vi "Amplifier Output Test Interface.vi"() -> ()   [LabVIEW 2012]
panel:
  out "Power Spectrum / PSD [Filtered]":cluster{"f0":dbl, "df":dbl, "magnitude":dbl[]}(graph)
  out "Signal [Filtered]":waveform(dbl)(graph)
  out "Power Spectrum / PSD [Non Filtered]":cluster{"f0":dbl, "df":dbl, "magnitude":dbl[]}(graph)
  out "Signal [Non Filtered]":waveform(dbl)(graph)
  in  "Filter":T1
  in  "Signal Acquisition":T2 {"Scale Type" items=["Volts"=10348, "Custom Scale"=10065]; "Sample Mode" items=["Finite Samples"=10178, "Continuous Samples"=10123, "Hardware Timed Single Point"=12522]; "Terminal Configuration" items=["Default"=-1, "RSE"=10083, "Differential"=10106, "Pseudodifferential"=12529]}
  in  "error in":errorcluster
  out "error out":errorcluster
  in  "Exit":bool caption="Start 2"
  in  "Filter":bool caption="Start 2"
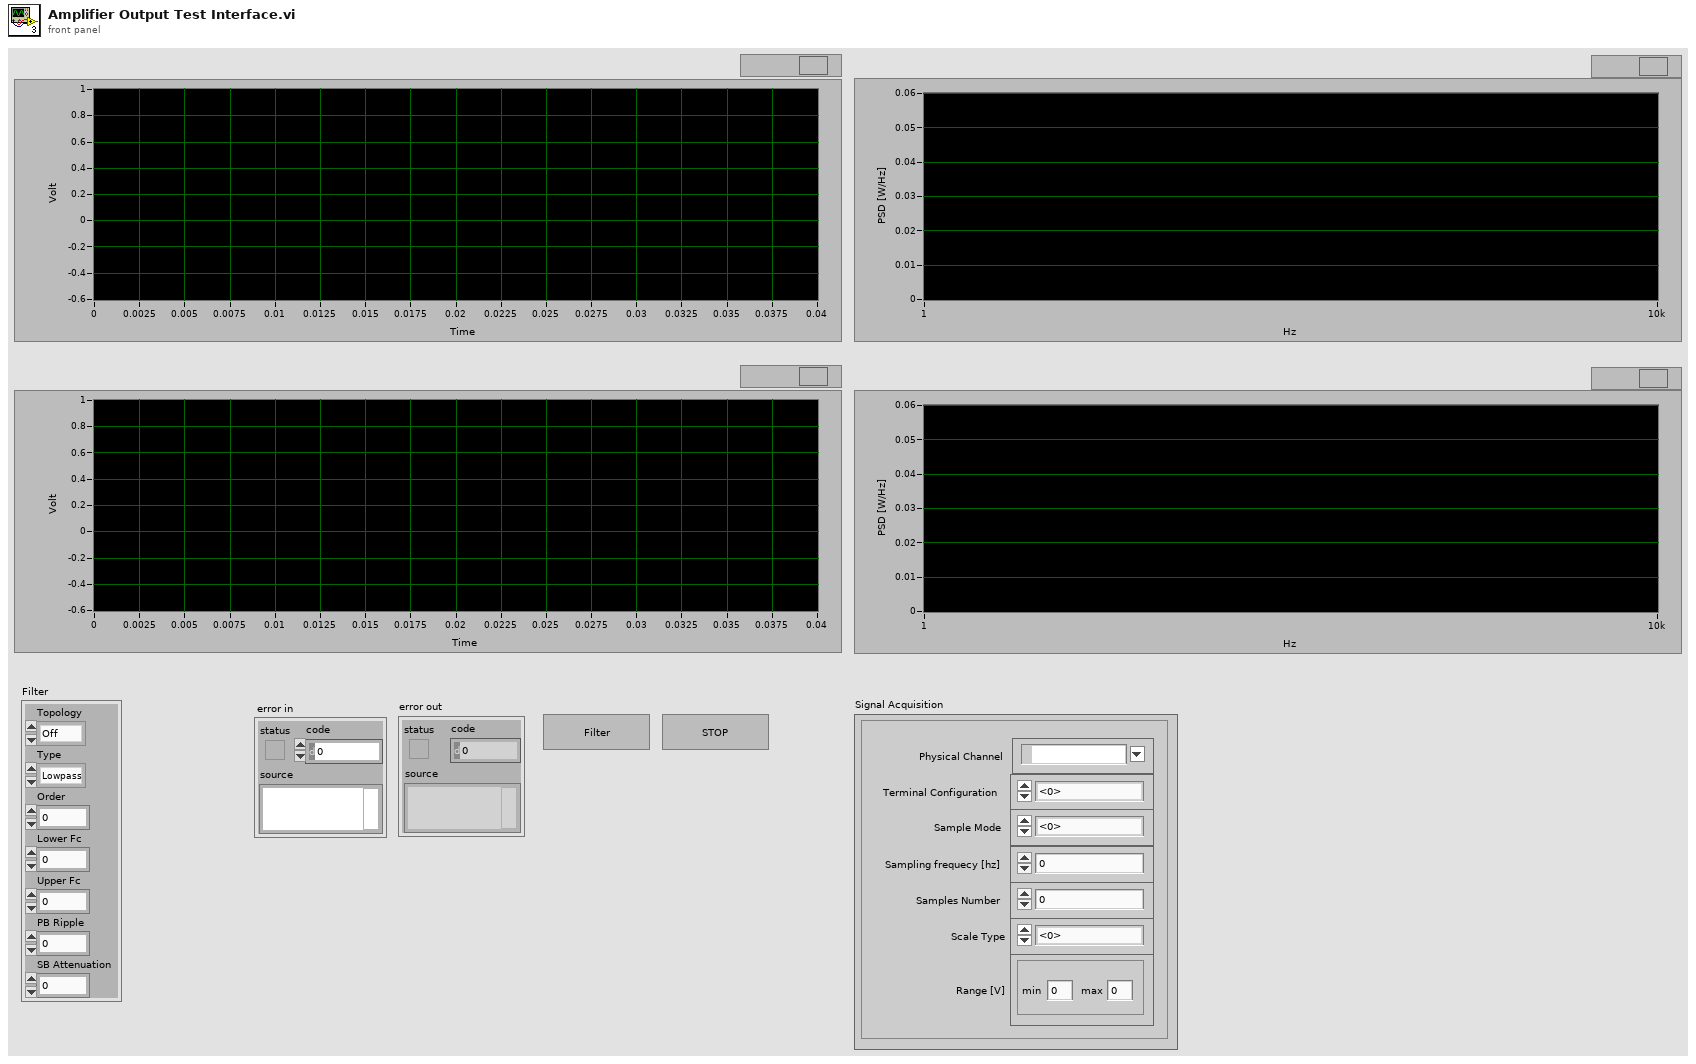
[diagram p1: front panel]
types:
  T1 = cluster{"Topology":enum16{"Off", "Butterworth", "Chebyshev", "Inverse Chebyshev", "Elliptic", "Bessel"}, "Type":enum16{"Lowpass", "Highpass", "Bandpass", "Bandstop"}, "Order":i32, "Lower Fc":dbl, "Upper Fc":dbl, "PB Ripple":dbl, "SB Attenuation":dbl}
  T2 = cluster{"Physical Channel":tag, "Terminal Configuration":i32, "Sample Mode":i32, "Scale Type":i32, "Range [V]":cluster{"max":dbl, "min":dbl}, "Sampling frequecy [hz]":dbl, "Samples Number":i32}
  T3 = cluster{"Signal [Filtered]":refnum<vi>, "Power Spectrum / PSD [Filtered]":refnum<vi>}
  T4 = cluster{"Signal [Non Filtered]":refnum<vi>, "Power Spectrum / PSD [Non Filtered]":refnum<vi>}
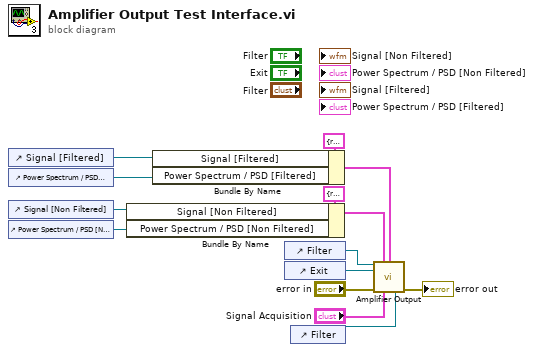
[diagram p0: block diagram]
diagram:
  n1 = control-ref of="Signal [Filtered]"() -> (w4:refnum<vi>)
  n2 = control-ref of="Power Spectrum / PSD [Filtered]"() -> (w3:refnum<vi>)
  n3 = control-ref of="Signal [Non Filtered]"() -> (w7:refnum<vi>)
  n4 = control-ref of="Power Spectrum / PSD [Non Filtered]"() -> (w6:refnum<vi>)
  n5 = Bundle By Name(cluster=T4 {"Signal [Non Filtered]"=refnum, "Power Spectrum / PSD [Non Filtered]"=refnum} ("Non Filtered"), "Signal [Non Filtered]"=w7, "Power Spectrum / PSD [Non Filtered]"=w6) -> (w2:T4)
  n6 = Bundle By Name(cluster=T3 {"Signal [Filtered]"=refnum, "Power Spectrum / PSD [Filtered]"=refnum} ("Filtered"), "Signal [Filtered]"=w4, "Power Spectrum / PSD [Filtered]"=w3) -> (w1:T3)
  n7 = control-ref of="Filter"() -> (w12:refnum<vi>)
  n8 = control-ref of="Exit"() -> (w11:refnum<vi>)
  n9 = control-ref of="Filter"() -> (w10:refnum<vi>)
  n10 = call "Amplifier Output.vi"("Filter"=w12, 1:w2, "Filtered"=w1, "Filter Led Indicator"=w11, "error in"="error in", "Signal Acquisition"="Signal Acquisition", "Exit"=w10) -> ("error out"=→"error out":errorcluster)  [unwired: 8 in]
